vi "Send New Data (Array).vi"(8 "error in (no error)":errorcluster, 9 "Timestamps (Now)":dbl[](array[numeric]), 10 "Data":dbl[](array[numeric]), 11 "MessageQ":refnum<class "MessageQ.lvclass">) -> (0 "error out":errorcluster)   [LabVIEW 2020, in "VolatusData.lvlib"]
uses:
  VolatusData.lvlib
  Volatus/MessageQ/MessageQ.lvclass
  New Data.ctl
  Volatus/MessageQ/MessageQ.lvclass/MessageQ.ctl
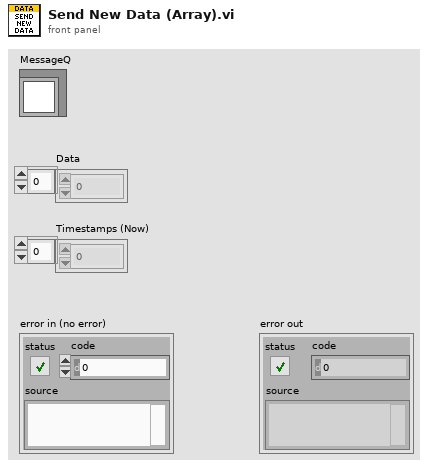
[diagram p1: front panel]
types:
  T1 = typedef "VolatusData.lvlib/New Data.ctl" = cluster{"Channels":waveform(dbl)[]}
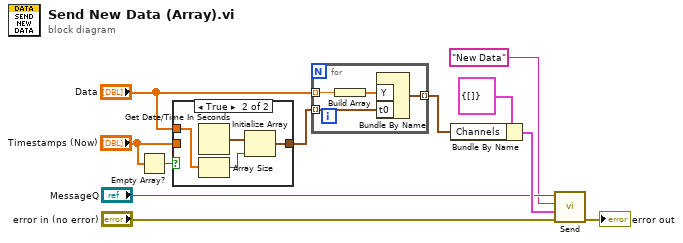
[diagram p0: block diagram]
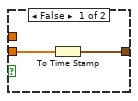
[diagram p2: hidden frame]
diagram:
  n1 = Empty Array?(array="Timestamps (Now)") -> (empty?=w2:bool)
  n2 = case shown="True" w2 {
    tunnel: [w13 w16] -> w5
    tunnel: "Timestamps (Now)" -> [w12 _]
    tunnel: "Data" -> [_ w15]
    frame False {
      n3 = To Time Stamp(1:w12) -> (0:w13:timestamp[])
    }
    frame True {
      n4 = Get Date/Time In Seconds() -> (seconds since 1Jan1904=w17:timestamp)
      n5 = Array Size(array=w15) -> (size(s)=w14:i32)
      n6 = Initialize Array(w17, w14) -> (w16:timestamp[])
    }
  }
  n7 = for {
    tunnel: w5 -> [w21] mode=indexing
    tunnel: "Data" -> [w20] mode=indexing
    tunnel: [w18] -> w4 mode=indexing
    n8 = Build Array(w20) -> (w19:dbl[])
    n9 = Bundle By Name("Y"=w19, "t0"=w21) -> (w18:waveform(dbl))  [unwired: 1 in]
  }
  n10 = Bundle By Name(cluster=T1 {"Channels"=[]} ("New Data"), "Channels"=w4) -> (w9:T1)
  n11 = call "Send.vi"("error in (no error)"="error in (no error)", "Data"=w9, "ID"="New Data", "MessageQ in"="MessageQ") -> ("error out"=→"error out":errorcluster)  [unwired: 6 in, 1 out]
